vi "VIsReplaceFailed.vi"() -> ()   [LabVIEW 2016, in "SwitchDependenciesVariables.lvlib"]
uses:
  SwitchDependenciesVariables.lvlib
panel:
  in  "VIsReplaceFailed":string
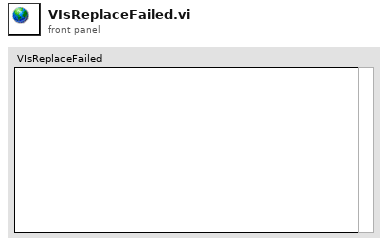
[diagram p1: front panel]
diagram:
